vi "KalmanFilter_changeL.vi"(1 "L":dbl[](array[numeric]), 6 "KalmanFilterVar":T1={"A"=[[1.0, 1.0], [0.0, 1.0]], "B"=[0.0, 1.0], "P0"=[[1.0, 0.0], [0.0, 1.0]], "C"=[1.0, 0.0], "Q"=[[1.0, 0.0], [0.0, 1.0]], "R"=1.0, "x0"=[0.0, 0.0]}, 10 "y":dbl, 11 "u":dbl) -> (2 "yhat":dbl, 3 "xhat":dbl[](array[numeric]))   [LabVIEW 2010, in "kevLib2011.lvlib"]
uses:
  kevLib2011.lvlib
  <vilib>/Analysis/NI_AALBase.lvlib
  <vilib>/Analysis/baseanly.llb/Real Dot Product.vi
  <vilib>/Analysis/baseanly.llb/A x Vector.vi
  <vilib>/Analysis/Matrix/Datatypes/RealMatrix.ctl
  <vilib>/Analysis/Matrix/NI_Matrix.lvlib
  KalmanFilterVar.ctl
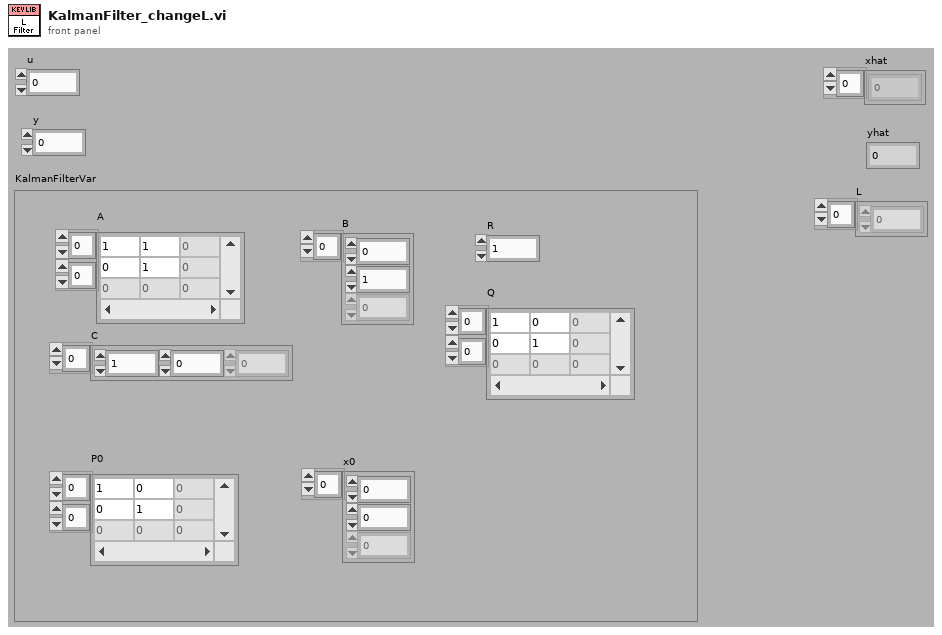
[diagram p1: front panel]
types:
  T1 = typedef "kevLib2011.lvlib/KalmanFilterVar.ctl" = cluster{"A":T2, "B":dbl[], "P0":T2, "C":dbl[], "Q":T2, "R":dbl, "x0":dbl[]}
  T2 = typedef "NI_Matrix.lvlib/RealMatrix.ctl" = dbl[][]
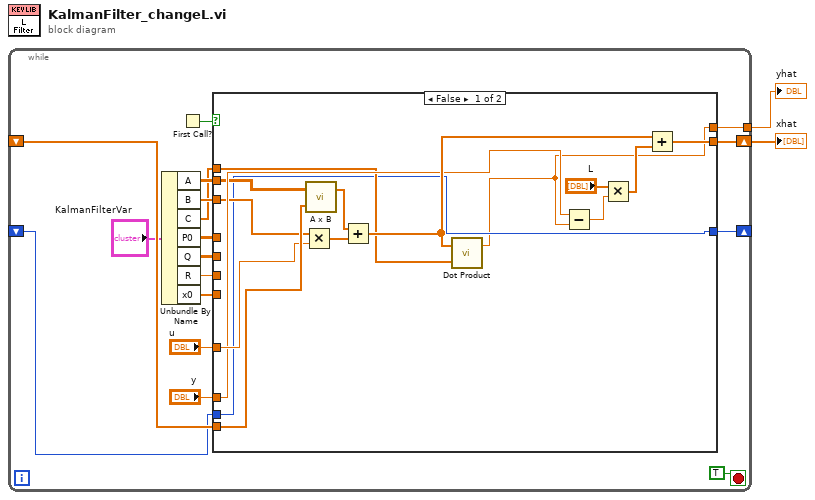
[diagram p0: block diagram]
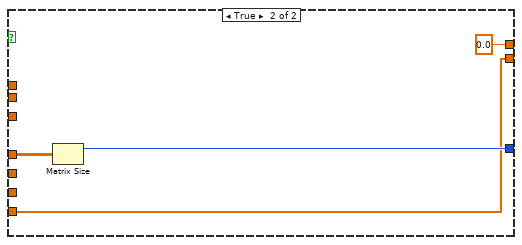
[diagram p2: hidden frame]
diagram:
  n1 = while {
    shift-right: [w18] -> w2
    shift-left: _ -> [w17]
    shift-right: [w13] -> _
    shift-left: _ -> [w12]
    tunnel: [w3] -> w1
    stop <- TRUE stop-if-true
    n2 = Unbundle By Name("KalmanFilterVar") -> ("A"=w10:T2, "B"=w9:dbl[], "C"=w4:dbl[], "P0"=w5:T2, "Q"=w8:T2, "R"=w7:dbl, "x0"=w6:dbl[])
    n3 = First Call?() -> (First Call?: T/F=w19:bool)
    n4 = case shown="False" w19 {
      tunnel: [w26 w35] -> w18
      tunnel: w17 -> [w34 _]
      tunnel: "u" -> [w33 _]
      tunnel: "y" -> [w29 _]
      tunnel: w12 -> [w22 _]
      tunnel: w8 -> [_ _]
      tunnel: w7 -> [_ _]
      tunnel: [w22 w38] -> w13
      tunnel: w9 -> [w25 _]
      tunnel: w10 -> [w24 _]
      tunnel: w4 -> [w23 _]
      tunnel: w5 -> [_ w37]
      tunnel: w6 -> [_ w35]
      tunnel: [w21 0.0 ("X * Y")] -> w3
      frame False {
        n5 = Multiply(x=w25, y=w33) -> (x*y=w31:dbl[])
        n6 = call-poly <vilib>:"A x B.vi"("Vector"=w34, "A"=w24) -> ("A x Vector"=w32:dbl[])  [unwired: 1 out]
        n7 = Add(x=w32, y=w31) -> (x+y=w30:dbl[])
        n8 = call-poly <vilib>:"Dot Product.vi"("Y Vector"=w23, "X Vector"=w30) -> ("X * Y"=w21:dbl)  [unwired: 1 out]
        n9 = Subtract(x=w29, y=w21) -> (x-y=w28:dbl)
        n10 = Multiply ("Multiply.vi")(x="L", y=w28) -> (x*y=w27:dbl[])
        n11 = Add ("Add.vi")(x=w30, y=w27) -> (x+y=w26:dbl[])
      }
      frame True {
        n12 = Matrix Size(0:w37) -> (1:w38:i32)  [unwired: 1 out]
      }
    }
  }
  "xhat" <- w2
  "yhat" <- w1
